vi "New Redis TCP Client.vi"(8 "error in (no error)":errorcluster, 9 "timeout ms (25000)":i32=25000, 10 "remote port or service name":u16=6379, 11 "address":string) -> (0 "error out":errorcluster, 3 "Redis TCP Client out":refnum<class "Redis TCP Client.lvclass">)   [LabVIEW 2019, in "Redis Client for LabVIEW.lvlib" / "Redis TCP Client.lvclass"]
uses:
  Redis TCP Client.lvclass
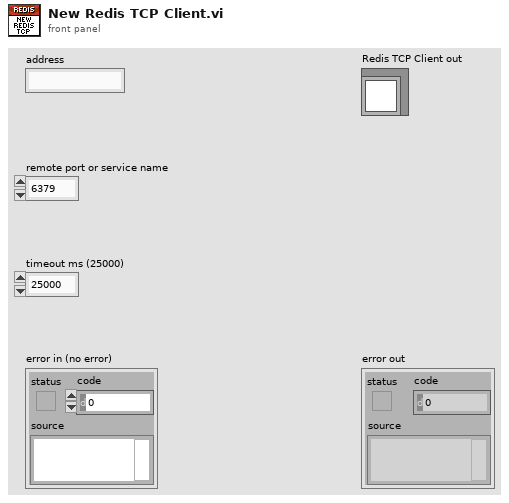
[diagram p1: front panel]
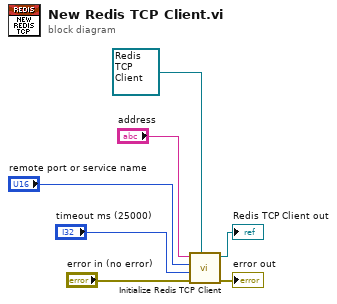
[diagram p0: block diagram]
diagram:
  n1 = call-dynamic "Initialize Redis TCP Client.vi"("Redis TCP Client in"=refnum<class "Redis TCP Client.lvclass"> refnum, "error in (no error)"="error in (no error)", "timeout ms (25000)"="timeout ms (25000)", "remote port or service name"="remote port or service name", "address"="address") -> ("error out"=→"error out":errorcluster, "Redis TCP Client out"=→"Redis TCP Client out":refnum<class "Redis TCP Client.lvclass">)  [unwired: 5 in]
